vi "blue puzzle.vi"() -> ()   [LabVIEW 2019]
uses:
  Program Files (x86)/National Instruments/LabVIEW 2019/project/EN1Course-master (12)/EN1Course-master/_Subs/SystemLink/SL_Subs/SL_XControl.xctl
  Program Files (x86)/National Instruments/LabVIEW 2019/project/EN1Course-master (12)/EN1Course-master/_Subs/SystemLink/SL_Subs/SystemLink_Write_String.vi
  <vilib>/httpClient/LabVIEWHTTPClient.lvlib
panel:
  in  "puzzle type 4":T1(xcontrol)={"Tag"="Puzzle Type", "Type"="STRING", "Data"=""}
  in  "puzzle type 3":T1(xcontrol)={"Tag"="Puzzle Type", "Type"="STRING", "Data"=""}
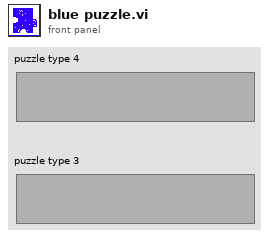
[diagram p1: front panel]
types:
  T1 = cluster{"Tag":string, "Type":string, "Data":string}
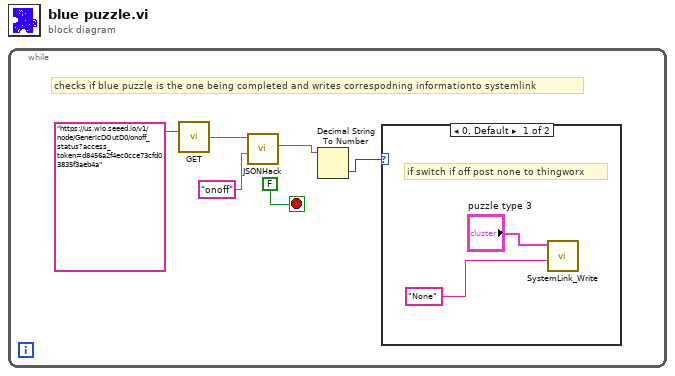
[diagram p0: block diagram]
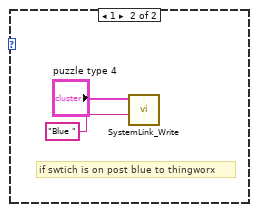
[diagram p2: hidden frame]
diagram:
  n1 = while {
    stop <- FALSE stop-if-true
    # "checks if blue puzzle is the one being completed and writes correspodning informationto systemlink"
    n2 = call <vilib>:"GET.vi"("url"="https://us.wio.seeed.io/v1/node/GenericDOutD0/onoff_status?access_token=d8456a2f4ec0cce73cfd03835f3aeb4a") -> ("body"=w4:string)  [unwired: 11 in, 3 out]
    n3 = call "JSONHack.vi"("search name"="onoff", "JSON in"=w4) -> ("Property (str)"=w2:string)  [unwired: 6 in, 3 out]
    n4 = Decimal String To Number(string=w2) -> (number=w1:i32)  [unwired: 2 in, 1 out]
    n5 = case shown="0, Default" w1 {
      frame 0, Default {
        # "if switch if off post none to thingworx"
        n6 = call-poly "SystemLink_Write.vi"("String"="None", "SL_XControl"="puzzle type 3") -> ()  [unwired: 10 in]
      }
      frame 1 {
        # "if swtich is on post blue to thingworx"
        n7 = call-poly "SystemLink_Write.vi"("String"="Blue ", "SL_XControl"="puzzle type 4") -> ()  [unwired: 10 in]
      }
    }
  }
